vi "CalculateRobotGroundVelocity.vi"(3 "Robot Heading (deg)":dbl, 4 "Velocity Y (ft/s)":dbl, 5 "Velocity X (ft/s)":dbl) -> (1 "Velocity Magnitude (ft/s)":dbl, 2 "Velocity Heading (deg)":dbl)   [LabVIEW 2020]
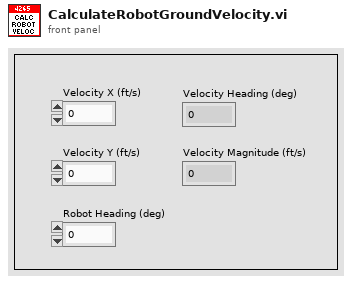
[diagram p1: front panel]
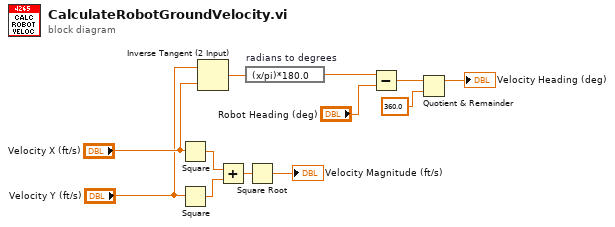
[diagram p0: block diagram]
diagram:
  n1 = Square(x="Velocity X (ft/s)") -> (x^2=w11:dbl)
  n2 = Square(x="Velocity Y (ft/s)") -> (x^2=w12:dbl)
  n3 = Inverse Tangent (2 Input)(1:"Velocity X (ft/s)", 2:"Velocity Y (ft/s)") -> (0:w9:dbl)
  n4 = Add(x=w11, y=w12) -> (x+y=w10:dbl)
  n5 = expression code="(x/pi)*180.0" "radians to degrees"(w9) -> (w8:dbl)
  n6 = Square Root(x=w10) -> (sqrt(x)=→"Velocity Magnitude (ft/s)":dbl)
  n7 = Subtract(x=w8, y="Robot Heading (deg)") -> (x-y=w6:dbl)
  n8 = Quotient & Remainder(x=w6, y=360.0) -> (x-y*floor(x/y)=→"Velocity Heading (deg)":dbl)  [unwired: 1 out]
